vi "SetDrawAreaSize.vi"(8 "error in (no error)":errorcluster, 11 "menu in":refnum<class "menu.lvclass">) -> (0 "error out":errorcluster, 3 "menu out":refnum<class "menu.lvclass">)   [LabVIEW 2009, in "menu.lvclass"]
uses:
  menu.lvclass
  menu.lvclass/menu.ctl
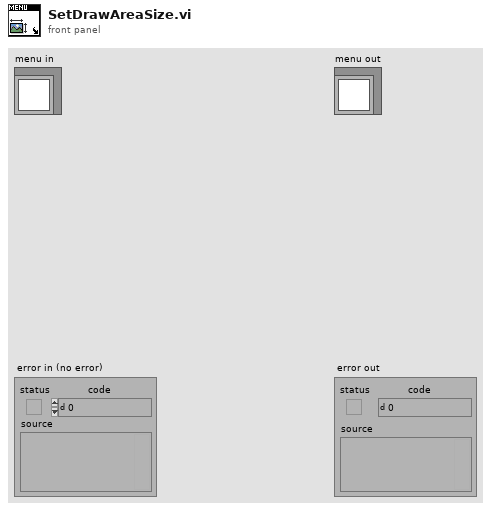
[diagram p1: front panel]
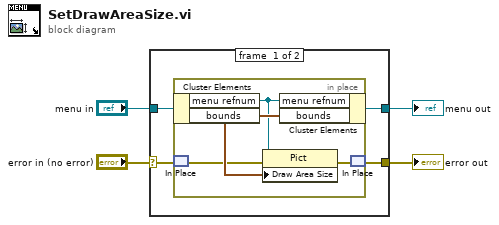
[diagram p0: block diagram]
diagram:
  n1 = case shown="No Error" "error in (no error)" {
    selector: "error in (no error)" -> [w5 w14]
    tunnel: [w6 w14] -> w1
    tunnel: [w7 w13] -> w3
    tunnel: "menu in" -> [w8 w13]
    frame #0 {
      n2 = in-place {
        n3 = in-place-cluster #1(w8) -> ("menu refnum"=w11:refnum<vi>, "bounds"=w12:cluster{"width":u32, "height":u32})
        n4 = in-place-match #2(w5) -> (w10:errorcluster)
        n5 = property class="Pict"(reference=w11, error in=w10, "Draw Area Size"=w12) -> (error out=w9:errorcluster)  [unwired: 1 out]
        n6 = in-place-cluster #1("menu refnum"=w11, "bounds"=w12) -> (w7:refnum<class "menu.lvclass">)
        n7 = in-place-match #2(w9) -> (w6:errorcluster)
      }
    }
    frame #1 {
    }
  }
  "menu out" <- w3
  "error out" <- w1
